vi "Test Process within App Log Info Message.vi"(8 "error in (no error)":errorcluster, 11 "Test Case In":refnum<class "Logger Test.lvclass">) -> (0 "error out":errorcluster, 3 "Test Case Out":refnum<class "Logger Test.lvclass">)   [LabVIEW 2020, in "Logger Test.lvclass"]
uses:
  Logger Test.lvclass
  C:/Program Files (x86)/National Instruments/LabVIEW 2020/vi.lib/Asteme/LUnit/Test Case.lvclass
  Mock Log Handler/Mock Log Handler.lvclass
  C:/Users/anton/Documents/GitHub/Triarc-Framework/source/Framework/Logging/Logging.lvclass
  Framework/Application/Application.lvclass
  C:/Users/anton/Documents/GitHub/Triarc-Framework/source/Framework/Process/Process.lvclass
  Mock Process/Mock Process.lvclass
  Framework/Process/Process.lvclass/Process.ctl
  Framework/Application/Application.lvclass/Application.ctl
  <vilib>/Asteme/LUnit/Test Case.lvclass/Test Case.ctl
  <vilib>/Asteme/LUnit/LUnit Assertion Result.lvclass/LUnit Assertion Result.ctl
  Framework/Process/Public/Lifecycle/Get Lifecycle State.vi
  Framework/Process/Protected/Messaging/Enqueue Message.vi
  Framework/Application/Private/Add Process to Map.vi
  Framework/Process/Protected/SubVIs/Set Context.vi
  Framework/Process/Private/SubVIs/Wait for finish.vi
  Framework/Process/Private/SubVIs/Set Lifecycle State.vi
  <vilib>/Asteme/LUnit/Palette/Pass.vi
  <vilib>/Asteme/LUnit/Palette/Fail.vi
  <vilib>/Asteme/LUnit/Variant to string.vi
  <vilib>/Asteme/LUnit/Set Assertion Type.vi
  <vilib>/AdvancedString/1D String Array to Delimited String.vi
  Framework/Process/Community/Leave Process Loop.vi
  <vilib>/Asteme/LUnit/Add test result.vi
  <vilib>/Asteme/LUnit/LUnit Write Passed.vi
  <vilib>/Asteme/LUnit/LUnit Get Test Case.vi
  <vilib>/Asteme/LUnit/LUnit Write Message.vi
  <vilib>/Asteme/LUnit/LUnit Write Description.vi
  <vilib>/Asteme/LUnit/LUnit Write Assertion Type.vi
  <vilib>/Asteme/LUnit/Read Test Case Name.vi
  <vilib>/Utility/error.llb/Error Cluster From Error Code.vi
  <vilib>/Asteme/LUnit/Assertion Result/LUnit Get Test Name.vi
  <vilib>/Utility/Data Type/Get Type Information.vi
  <vilib>/Utility/LVClass/Get LV Class Name.vi
  Framework/Process/Process.lvclass
  <vilib>/Asteme/LUnit/LUnit Assertion Result.lvclass
  Framework/Logging/Logging.lvclass
  <vilib>/Asteme/LUnit/Test Case.lvclass
  Support/Framework Test Support.lvlib
  C:/Users/anton/Documents/GitHub/Triarc-Framework/source/Framework/Base/Base.lvclass
  C:/Users/anton/Documents/GitHub/Triarc-Framework/source/Framework/Error Handler Interface/Error Handler Interface.lvclass
  C:/Users/anton/Documents/GitHub/Triarc-Framework/source/Framework/Application/Application.lvclass
  C:/Users/anton/Documents/GitHub/Triarc-Framework/source/Framework Test/Logger Test/Logger Test.lvclass
  C:/Users/anton/Documents/GitHub/Triarc-Framework/source/Framework Test/Mock Log Handler/Mock Log Handler.lvclass
  C:/Users/anton/Documents/GitHub/Triarc-Framework/source/Framework Test/Mock Process/Mock Process.lvclass
  C:/Users/anton/Documents/GitHub/Triarc-Framework/source/Framework/Helper Loop/Helper Loop.lvclass
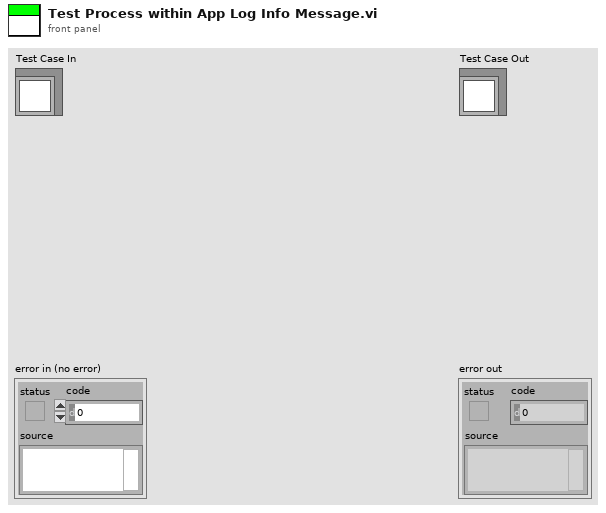
[diagram p1: front panel]
types:
  T1 = typedef "Mock Log Handler.lvclass/Log Entry.ctl" = cluster{"Level":string, "Source":string, "Message":string}
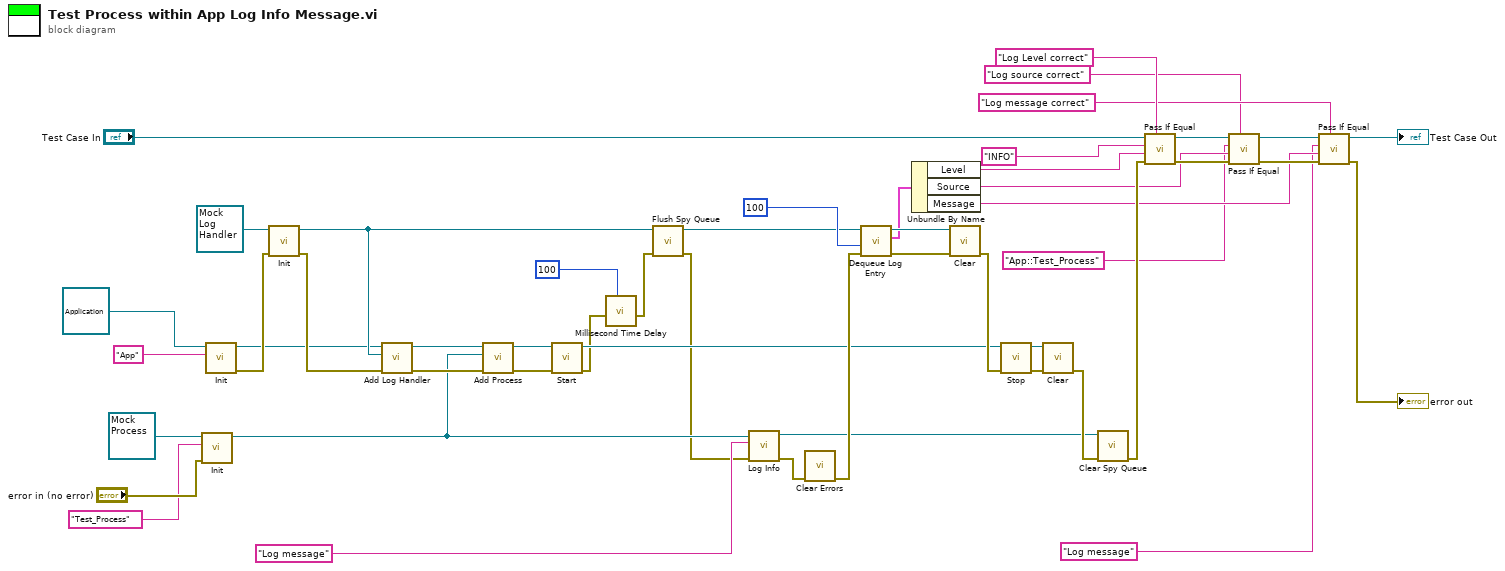
[diagram p0: block diagram]
diagram:
  n1 = call-dynamic "Init.vi"("error in (no error)"="error in (no error)", "Name"="Test_Process", "Mock Process In"=refnum<class "Mock Process.lvclass"> refnum) -> ("Mock Process Out"=w4:refnum<class "Mock Process.lvclass">)  [unwired: 7 in, 1 out]
  n2 = call-dynamic "Init.vi"("Name"="App", "Process In"=refnum<class "Application.lvclass"> refnum ("Application.lvclass")) -> ("error out"=w45:errorcluster, "Process Out"=w2:refnum<class "Application.lvclass">)  [unwired: 8 in]
  n3 = call-dynamic "Init.vi"("error in (no error)"=w45, "Mock Log Handler In"=refnum<class "Mock Log Handler.lvclass"> refnum ("Mock Log Handler.lvclass")) -> ("error out"=w44:errorcluster, "Mock Log Handler Out"=w9:refnum<class "Mock Log Handler.lvclass">)  [unwired: 8 in]
  n4 = call "Add Log Handler.vi"("error in (no error)"=w44, "Log Handler"=w9, "Process In"=w2) -> ("error out"=w19:errorcluster, "Process Out"=w18:refnum<class "Application.lvclass">)  [unwired: 7 in]
  n5 = call "Add Process.vi"("error in (no error)"=w19, "Process"=w4, "Rig In"=w18) -> ("error out"=w15:errorcluster, "Rig Out"=w1:refnum<class "Application.lvclass">)  [unwired: 7 in]
  n6 = call "Start.vi"("error in (no error)"=w15, "Process In"=w1) -> ("error out"=w7:errorcluster, "Process Out"=w11:refnum<class "Application.lvclass">)  [unwired: 8 in]
  n7 = call "Millisecond Time Delay.vi"("milliseconds to wait"=u32 100, "error in (no error)"=w7) -> ("error out"=w6:errorcluster)  [unwired: 7 in]
  n8 = call "Flush Spy Queue.vi"("error in (no error)"=w6, "Mock Log Handler in"=w9) -> ("error out"=w3:errorcluster, "Mock Log Handler out"=w8:refnum<class "Mock Log Handler.lvclass">)  [unwired: 7 in, 1 out]
  n9 = call "Log Info.vi"("error in (no error)"=w3, "Message"="Log message", "Logging In"=w4) -> ("error out"=w25:errorcluster, "Logging Out"=w12:refnum<class "Mock Process.lvclass">)  [unwired: 7 in]
  n10 = call <vilib>:"Clear Errors.vi"("error in (no error)"=w25) -> ("error out"=w24:errorcluster)  [unwired: 5 in, 1 out]
  n11 = call "Dequeue Log Entry.vi"("error in (no error)"=w24, "timeout in ms (-1)"=100, "Mock Log Handler in"=w8) -> ("error out"=w42:errorcluster, "Entry"=w39:T1, "Mock Log Handler out"=w43:refnum<class "Mock Log Handler.lvclass">)  [unwired: 5 in, 1 out]
  n12 = Unbundle By Name(w39) -> ("Level"=w38:string, "Source"=w28:string, "Message"=w27:string)
  n13 = call-dynamic "Clear.vi"("error in (no error)"=w42, "Mock Log Handler In"=w43) -> ("error out"=w40:errorcluster)  [unwired: 8 in, 1 out]
  n14 = call "Stop.vi"("error in (no error)"=w40, "Process In"=w11) -> ("error out"=w14:errorcluster, "Process Out"=w13:refnum<class "Application.lvclass">)  [unwired: 7 in, 1 out]
  n15 = call-dynamic "Clear.vi"("error in (no error)"=w14, "Application In"=w13) -> ("error out"=w47:errorcluster)  [unwired: 8 in, 1 out]
  n16 = call-dynamic "Clear Spy Queue.vi"("error in (no error)"=w47, "Mock Process In"=w12) -> ("error out"=w32:errorcluster)  [unwired: 8 in, 1 out]
  n17 = call <vilib>:"Pass If Equal.vi"("Description"="Log Level correct", "error in (no error)"=w32, "Actual"=w38, "Expected"="INFO", "Test Case In"="Test Case In") -> ("error out"=w34:errorcluster, "Test Case Out"=w49:refnum<class "Logger Test.lvclass">)  [unwired: 5 in]
  n18 = call <vilib>:"Pass If Equal.vi"("Description"="Log source correct", "error in (no error)"=w34, "Actual"=w28, "Expected"="App::Test_Process" ("Name"), "Test Case In"=w49) -> ("error out"=w33:errorcluster, "Test Case Out"=w36:refnum<class "Logger Test.lvclass">)  [unwired: 5 in]
  n19 = call <vilib>:"Pass If Equal.vi"("Description"="Log message correct", "error in (no error)"=w33, "Actual"=w27, "Expected"="Log message" ("Message"), "Test Case In"=w36) -> ("error out"=→"error out":errorcluster, "Test Case Out"=→"Test Case Out":refnum<class "Logger Test.lvclass">)  [unwired: 5 in]
